vi "Robot Global Data.vi"() -> ()   [LabVIEW 2012]
doc: "This global VI can contain as many global variables as you need. Place a control on the panel, give it a good name. To read or write to it from a VI, drag the icon to the diagram of that VI. You can also drag from the project. Click on the node to change which global you access. You shouldn't have multiple locations writing to a global or it will cause a race-condition."
uses:
  <vilib>/Rock Robotics/WPI/Camera/WPI_CameraImageSize.ctl
  <vilib>/Rock Robotics/WPI/DriverStation/WPI_DriverStationRobotMode2.ctl
  <vilib>/Rock Robotics/WPI/Relay/WPI_RelayValue.ctl
panel:
  out "ShootOutHarvestor":T1
  out "ShootOutFlipper2":dbl
  in  "PTO Disabled":dbl=100.0
  in  "PTO Enabled":dbl=135.0
  out "ShootOutWheelB":dbl
  in  "ShootWheelBSpd":dbl=0.7
  out "ClimbOutDep":dbl
  out "ClimbOutExt":dbl
  in  "ClimbConst":T2
  in  "ClimbCase":dbl
  in  "ClimbDepEnable":bool
  in  "ClimbFoldEnable":bool
  in  "ClimbExtEnable":bool
  in  "ClimbRetEnable":bool
  in  "ClimbManualDep":dbl
  in  "ClimbManualExt":dbl
  out "Current File":dbl
  out "Circle Info":cluster{dbl, dbl}
  out "ShootOutFlipper":dbl
  out "ShootOutRollers":dbl
  out "ShootOutWheelF":dbl
  out "ShootOutElev":dbl
  out "ShootOutIndexer":dbl
  in  "ShootTrackEnable":bool
  in  "ShootStartWheels":bool
  in  "ShootIndexerEnable":bool
  in  "ShootCase":dbl
  in  "ShootManualElev":dbl
  in  "ShootIndexerSpd":dbl=0.5
  in  "ShootWheelFSpd":dbl=0.85
  in  "ShootConstElev":T3={"Ground"=4.0, "1"=3.0, "2"=2.5, "3"=2.5, "4"=2.5}
  in  "ShootRollerSpd":dbl
  in  "ShootConstFlipper":T4={"Down 1"=0.2, "Up 1"=0.8, "Up 2"=0.8, "Down 2"=0.2}
  out "Target Info":cluster{"X":dbl, "Y":dbl, "Distance (ft)":dbl}
  in  "Servo Positions":T5={"Right Servo High"=75.0, "Right Servo Mid"=92.0, "Right Servo Low"=110.0, "Left Servo High"=55.0, "Left Servo Mid"=75.0, "Left Servo Low"=90.0}
  out "Auton Array":dbl[][](array[numeric]) format="%0.3f"
  out "Auton Files":string[](array[string])
  out "Number of Auton Files":dbl
  in  "Robot Mode":T6
  in  "LED toggle rate (ms)":u32=20
  in  "image size":T7=enum."160x120"
  in  "Enable Vision":bool=TRUE
  # "Shoot Globals"
  # "Climber Globals"
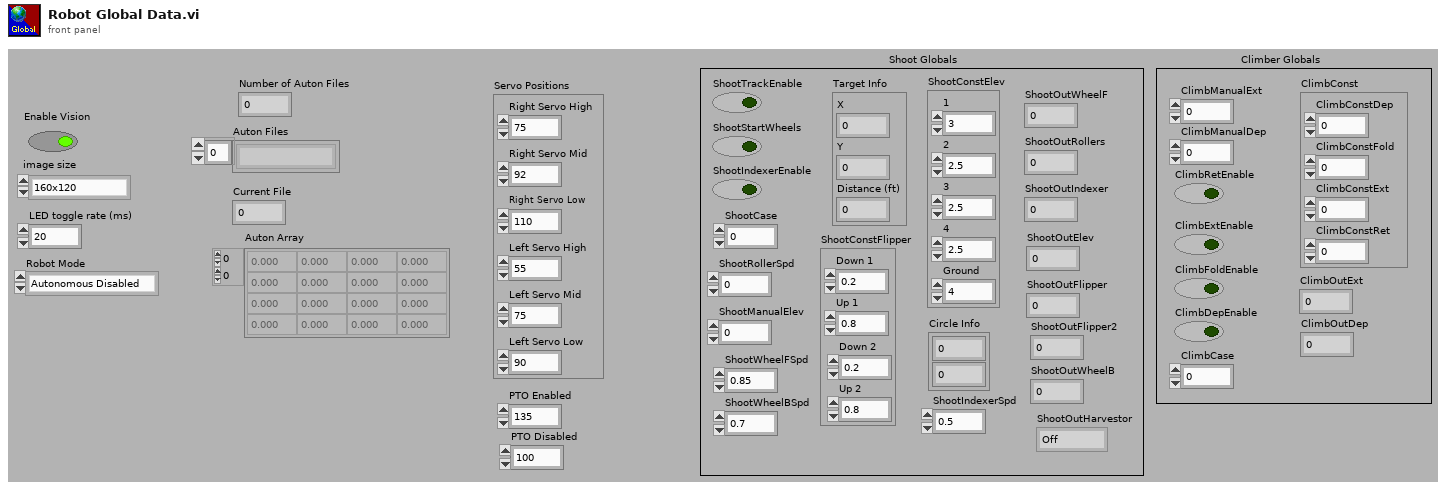
[diagram p1: front panel]
types:
  T1 = typedef "WPI_RelayValue.ctl" = enum16{"Off", "On", "Forward", "Reverse"}
  T2 = cluster{"ClimbConstDep":dbl, "ClimbConstFold":dbl, "ClimbConstExt":dbl, "ClimbConstRet":dbl}
  T3 = cluster{"Ground":dbl, "1":dbl, "2":dbl, "3":dbl, "4":dbl}
  T4 = cluster{"Down 1":dbl, "Up 1":dbl, "Up 2":dbl, "Down 2":dbl}
  T5 = cluster{"Right Servo High":dbl, "Right Servo Mid":dbl, "Right Servo Low":dbl, "Left Servo High":dbl, "Left Servo Mid":dbl, "Left Servo Low":dbl}
  T6 = typedef "WPI_DriverStationRobotMode2.ctl" = enum16{"Autonomous Disabled", "Autonomous Enabled", "Teleop Disabled", "Teleop Enabled", "Timeout", "Finish", "Test Disabled", "Test Enabled"}
  T7 = typedef "WPI_CameraImageSize.ctl" = enum16{"640x480", "320x240", "160x120"}
diagram:
